vi "LVClass_DataClient dtor.vi"(0 "DataClient in":refnum<class "DataClient.lvclass">, 11 "error in (no error)":errorcluster) -> (4 "DataClient out":refnum<class "DataClient.lvclass">, 15 "error out":errorcluster)   [LabVIEW 2020, in "DataClient.lvclass"]
doc: "Client destructor.\n\n<B>clientIn</B> : Client object.\n<B>clientOut</B> : Client object."
uses:
  DataClient.lvclass
  DataClient.lvclass/DataClient.ctl
  ClientServerDataID.ctl
  ClientServerDataType.ctl
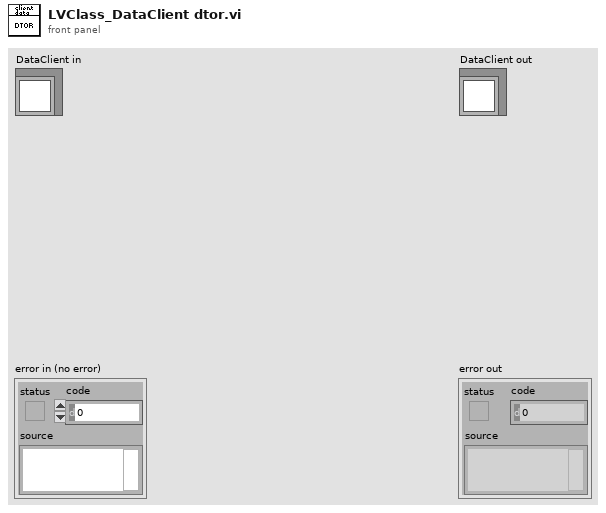
[diagram p1: front panel]
types:
  T1 = typedef "ClientServerDataID.ctl" = cluster{"Name":string, "Type":T2}
  T2 = typedef "ClientServerDataType.ctl" = enum16{"Boolean", "Integer", "Float", "String", "HasoSlopes", "Image"}
  T3 = typedef "Handle creation.ctl" = enum16{"By ctor", "By write function"}
  T4 = typedef "ClassID.ctl" = i64
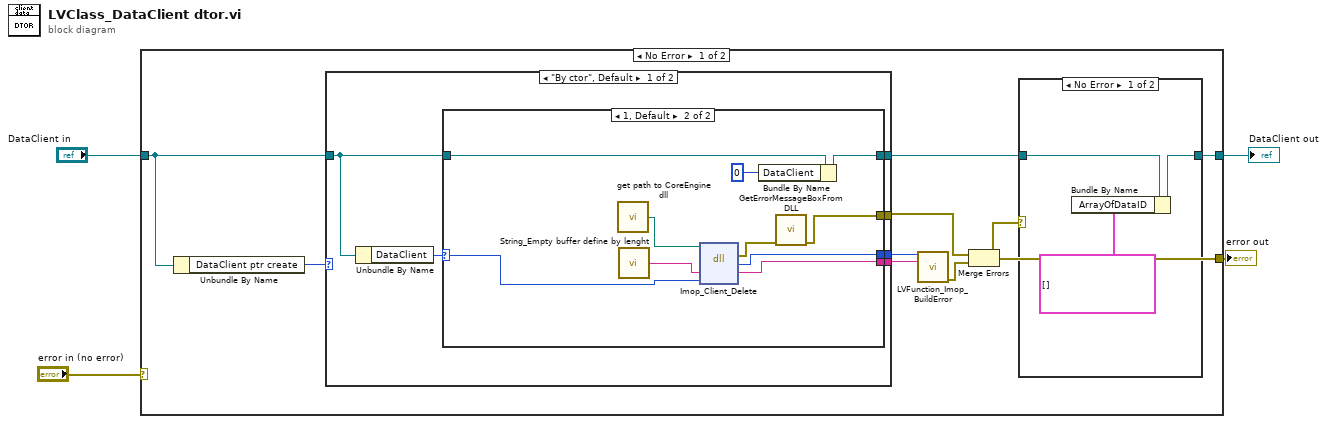
[diagram p0: block diagram]
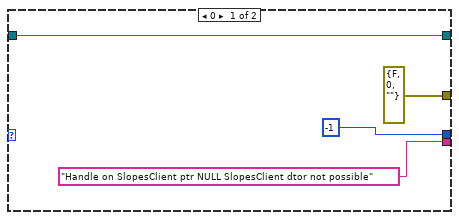
[diagram p3: hidden frame]
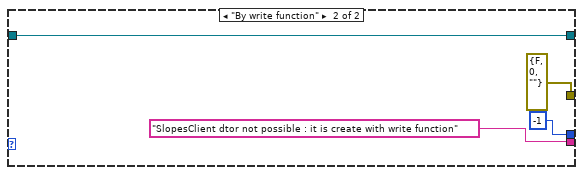
[diagram p4: hidden frame]
diagram:
  n1 = case shown="No Error" "error in (no error)" {
    selector: "error in (no error)" -> [_ w43]
    tunnel: [w7 w43] -> w3
    tunnel: [w6 w42] -> w1
    tunnel: "DataClient in" -> [w8 w42]
    frame No Error {
      n2 = Unbundle By Name(w8) -> ("DataClient ptr create"=w11:T3)
      n3 = case shown="\"By ctor\", Default" w11 {
        tunnel: [w23 "SlopesClient dtor not possible : it is create with write function" ("message")] -> w13
        tunnel: [w22 -1] -> w12
        tunnel: [w21 w39] -> w5
        tunnel: w8 -> [w20 w39]
        tunnel: [w18 errorcluster {"status"=FALSE, "code"=0, "source"=""} ("error OUT")] -> w10
        frame "By ctor", Default {
          n4 = Unbundle By Name(w20) -> ("DataClient"=w19:T4)
          n5 = case shown="1, Default" w19 {
            selector: w19 -> [_ w34]
            tunnel: ["Handle on SlopesClient ptr NULL SlopesClient dtor not possible" ("message") w36] -> w23
            tunnel: [-1 w35] -> w22
            tunnel: w20 -> [w25 w31]
            tunnel: [w25 w30] -> w21
            tunnel: [errorcluster {"status"=FALSE, "code"=0, "source"=""} ("error OUT") w29] -> w18
            frame 0 {
            }
            frame 1, Default {
              n6 = call "get path to CoreEngine dll.vi"() -> ("path to wavekit library"=w33:path)  [unwired: 14 in, 1 out]
              n7 = call "String_Empty buffer define by lenght.vi"() -> ("Empty buffer"=w37:string)  [unwired: 1 in]
              n8 = dll-call lib="D:/soft/HASO_v3/SVN_trunk/ImOpCoreEngine4_LV2011/DLLs/c_interface_vc100.dll" fn="Imop_Client_Delete"(path in=w33, "message"=w37, "SlopesClient"=w34) -> (error out=w32:errorcluster, "return type"=w35:i32, "message"=w36:string)  [unwired: 3 in, 1 out]
              n9 = Bundle By Name(cluster=w31, "DataClient"=0 ("SlopesServer")) -> (w30:refnum<class "DataClient.lvclass">)
              n10 = call "GetErrorMessageBoxFromDLL.vi"("error IN"=w32) -> ("error OUT"=w29:errorcluster)  [unwired: 10 in]
            }
          }
        }
        frame "By write function" {
        }
      }
      n11 = call "LVFunction_Imop_BuildError.vi"("code"=w12, "String to Prepend to source (\"\")"=w13) -> ("error out"=w9:errorcluster)  [unwired: 13 in]
      n12 = Merge Errors(w10, w9) -> (w7:errorcluster)
      n13 = case shown="No Error" w7 {
        tunnel: [w14 w17] -> w6
        tunnel: w5 -> [w16 w17]
        frame No Error {
          n14 = Bundle By Name(cluster=w16, "ArrayOfDataID"=T1[] []) -> (w14:refnum<class "DataClient.lvclass">)
        }
        frame Error {
        }
      }
    }
    frame Error {
    }
  }
  "error out" <- w3
  "DataClient out" <- w1
